vi "Dashboard Main.vi"() -> ()   [LabVIEW 2020]
uses:
  <vilib>/event_ctls.llb/eventvkey.ctl
  <vilib>/Rock Robotics/Network Tables/NT Read Numeric Array.vi
  <vilib>/Rock Robotics/WPI/Dashboard/WPI_DashboardLogging Global.vi
panel:
  in  "Graph4":string="Number"
  in  "Graph3":string="Number"
  in  "Graph2":string="Number"
  in  "Graph1":string="Number"
  in  "Camera Settings Right":T1={"Frame Rate"=30, "Compression"=30, "Size"=1, "DB Camera Config"=FALSE} {"Frame Rate" scale=1.0..30.0; "Compression" scale=100.0..-1.0; "Size" items=["640x480", "320x240", "160x120"]}
  in  "Camera Name Right":string(combo)="No Camera Selection"
  out "Camera Perf":string
  in  "Camera Settings":T1={"Frame Rate"=30, "Compression"=30, "Size"=1, "DB Camera Config"=FALSE} {"Frame Rate" scale=1.0..30.0; "Compression" scale=100.0..-1.0; "Size" items=["640x480", "320x240", "160x120"]}
  in  "TCP":refnum<k5>
  in  "Rec Mode":enum32{"Stop", "Record", "Playback"}(radio)
  out "Robot IP":string
  out "Image Message":string="Timeout in Camera Communications"
  in  "Dashboard Tab":T2(tab)
  out "Waveform Graph":dbl[](graph)
  in  "Select Auto":string(combo)="Select Autonomous ..."
  out "NT Connection":bool
  out "Mode":T3(ring)=enum."Auto Disabled"
  out "Right Camera Perf":cluster{"Bandwidth (Mbps)":dbl, "FPS":dbl}
  out "Camera Image Right":T4(plugin-control)
  in  "DB/String 9":string
  in  "DB/String 8":string
  in  "DB/String 7":string
  in  "DB/String 6":string
  in  "DB/String 5":string
  in  "DB/String 4":string
  in  "DB/String 3":string
  in  "DB/String 2":string
  in  "DB/String 1":string
  in  "DB/String 0":string
  in  "DB/Slider 0":dbl(slide) scale=0.0..5.0
  in  "DB/Slider 1":dbl(slide) scale=0.0..5.0
  in  "DB/Slider 2":dbl(slide) scale=0.0..5.0
  in  "DB/Slider 3":dbl(slide) scale=0.0..5.0
  out "DB/LED 3":bool
  out "DB/LED 2":bool
  out "DB/LED 1":bool
  out "DB/LED 0":bool
  in  "DB/Button 3":bool
  in  "DB/Button 2":bool
  in  "DB/Button 1":bool
  in  "DB/Button 0":bool caption="New Name"
  in  "Test Slider":dbl(slide) scale=0.0..100.0 scale format="%#_3g"
  in  "On/Off":bool caption="Solenoid"
  in  "Test Name":u16(ring) items=["Select the test to run..."]
  in  "Test Tree":string(tree)
  in  "Motor":cluster{"Value":dbl, "Enable":bool} {"Value" scale=-1.0..1.0 scale format="%#_3g"}
  out "Progress":T5 {"Test Progress" scale=0.0..100.0}
  in  "Rev/Fwd":cluster{"Forward":bool, "Reverse":bool}
  in  "Test Ring":u16(ring) items=["Monochrome", "Color"]
  in  "CheckList":i32(listbox)
  out "Tree":string(tree)
  out "Camera Image":T4(plugin-control)
  out "Background":bool
  in  "Camera Name":string(combo)="No Camera Selection"
  # "HW"
  # "HW"
  # "This tab is a great place for autonomous settings and robot-specific values.\nPlace controls and indicators inside this tab and match name to\nDashboard Variables on robot. You can also delete this comment."
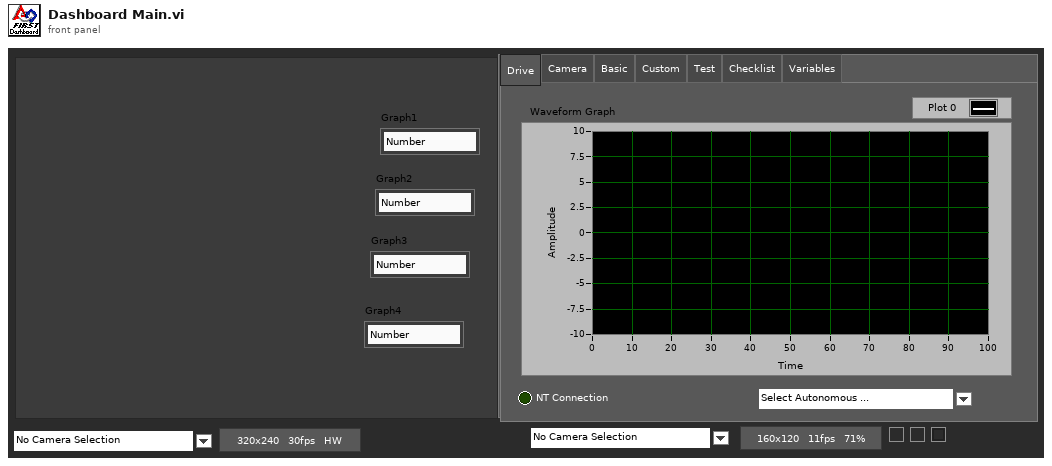
[diagram p1: front panel]
types:
  T1 = cluster{"Frame Rate":i32, "Compression":i32, "Size":u16, "DB Camera Config":bool}
  T2 = enum32{"Drive", "Camera", "Basic", "Custom", "Test", "Checklist", "Variables"}
  T3 = enum8{"Tele-Op Disabled", "Tele-Op Enabled", "Auto Disabled", "Auto Enabled", "Test Disabled", "Test Enabled", "Disconnected", "No Code", "E-Stop"}
  T4 = typedef "IMAQ Image.ctl" = refnum<image>
  T5 = cluster{"Test Progress":u8, "Test Progress Text":string}
  T6 = cluster{"Save Path":path, "Interval (s)":dbl, "Keep":i32}
  T7 = enum32{"Drive", "Camera", "Basic", "Custom", "Test", "Commands", "Checklist", "Variables"}
  T8 = typedef "Image Type" = u32
  T9 = cluster{"Error Strings":string, "Disable Counts":cluster{u16, u16}, "Rail Faults":cluster{u16, u16, u16}, "Robot IP":string, "DB Mode":u8, "Event Info":cluster{"Name":string, "Type":u8, "Number":u16, "Replay":u8}}
  T10 = cluster{"Storage":cluster{"Disk Free":u64, "RAM Block":u32, "RAM free":u32}, "CPU Utilization":cluster{"CPU % ISR":sgl, "CPU % Time Crit":sgl, "CPU % Timed Str":sgl, "CPU % High":sgl, "CPU % Above":sgl, "CPU % Normal":sgl, "CPU % Low":sgl}, "CAN":cluster{"% Bus Utilization":sgl, "Bus Off Cnt":u32, "TX_FIFO Full Cnt":u32, "Receive Error Cnt":u8, "Transmit Error Cnt":u8}, "HID":cluster{"HID Outputs":u32, "Rumble Low":u16, "Rumble High":u16}[]}
  T11 = cluster{"Status bits":cluster{"Test Mode":bool, "Autonomous":bool, "Enabled":bool, "Code Start":bool, "Brownout":bool, "Reserved 2":bool, "Reserved 3":bool, "E-Stop":bool}, "Code Trace":cluster{"Disabled":bool, "TeleOp":bool, "Auto":bool, "Test":bool}, "Controller Type":enum16{"unknown", "cRIO", "roboRio"}, "Code?":enum16{"unknown", "noCode", "code"}, "Battery V":dbl}
  T12 = cluster{"Control Bits":cluster{"TestMode":bool, "Autonomous":bool, "Enabled":bool, "FMS Present":bool, bool, bool, bool, "E-Stop":bool}, "Team Station ":u8, "Countdown":sgl, "Joystick Values":cluster{"Axes":dbl[], "Buttons":bool[], "POVs":i16[]}[]}
  T13 = cluster{"Axes":dbl[], "Buttons":bool[], "POVs":i16[]}[]
  T14 = cluster{"Axes":dbl[], "Buttons":bool[], "POVs":i16[]}
  T15 = cluster{"Camera Image":refnum<vi>, "Dashboard Tab":refnum<vi>, "Background":refnum<vi>, "Rec Mode":refnum<vi>, "Test Slider":refnum<vi>, "On/Off ":refnum<vi>, "Test Ring":refnum<vi>, "Rev/Fwd":refnum<vi>, "Test Name":refnum<vi>, "Motor":refnum<vi>, "Progress":refnum<vi>, "CheckList":refnum<vi>, "Tree":refnum<vi>, "Test Tree":refnum<vi>, "Camera Settings":refnum<vi>, "Camera Name":refnum<vi>, "Camera Perf":refnum<vi>, "Camera Settings Right":refnum<vi>, "Camera Name Right":refnum<vi>, "Camera Image Right":refnum<vi>}
  T16 = cluster{"Global Rectangle":i32[], "Contours":cluster{"Contour Type":u32, "ROI Type":u32, "Points":i32[]}[]}
  T17 = cluster{"Camera Name":string, string, "Saved DB Images Info":cluster{"Save Path":path, "Interval (s)":dbl, "Keep":i32}}
  T18 = cluster{"Camera Name Right":string, string, "Saved DB Images Info":cluster{"Save Path":path, "Interval (s)":dbl, "Keep":i32}}
  T19 = cluster{"Operation":enum16{"Update", "Clear"}, "Color Box":u32}[]
  T20 = typedef "eventvkey.ctl" = enum16{"ASCII", "Enter", "Return", "Shift", "Ctrl", "Alt", "Cmd", "Opt", "Caps", "NumLock", "Clear", "Break", "Up", "Down", "Left", "Right", "Insert", "Delete", "Home", "End", "PageUp", "PageDown", "Escape", "Help", "Pause", "ScrollLock", "F1", "F2", "F3", "F4", "F5", "F6", "F7", "F8", "F9", "F10", "F11", "F12", "F13", "F14", "F15", "F16", "F17", "F18", "F19", "F20", "F21", "F22", "F23", "F24", "Play", "VolumeUp", "VolumeDown", "Mute", "Two Byte Char"}
  T21 = cluster{"Image Size":bool, "Image Type":bool, "Pixel Value":bool, "ROI Information":bool, "Zoom Factor":bool}
  T22 = cluster{"Operation":enum16{"Update", "Clear"}, "Color Box":u32}
  T23 = cluster{"Shift":bool, "Ctrl":bool, "Alt":bool, "Cmd":bool, "Opt":bool}
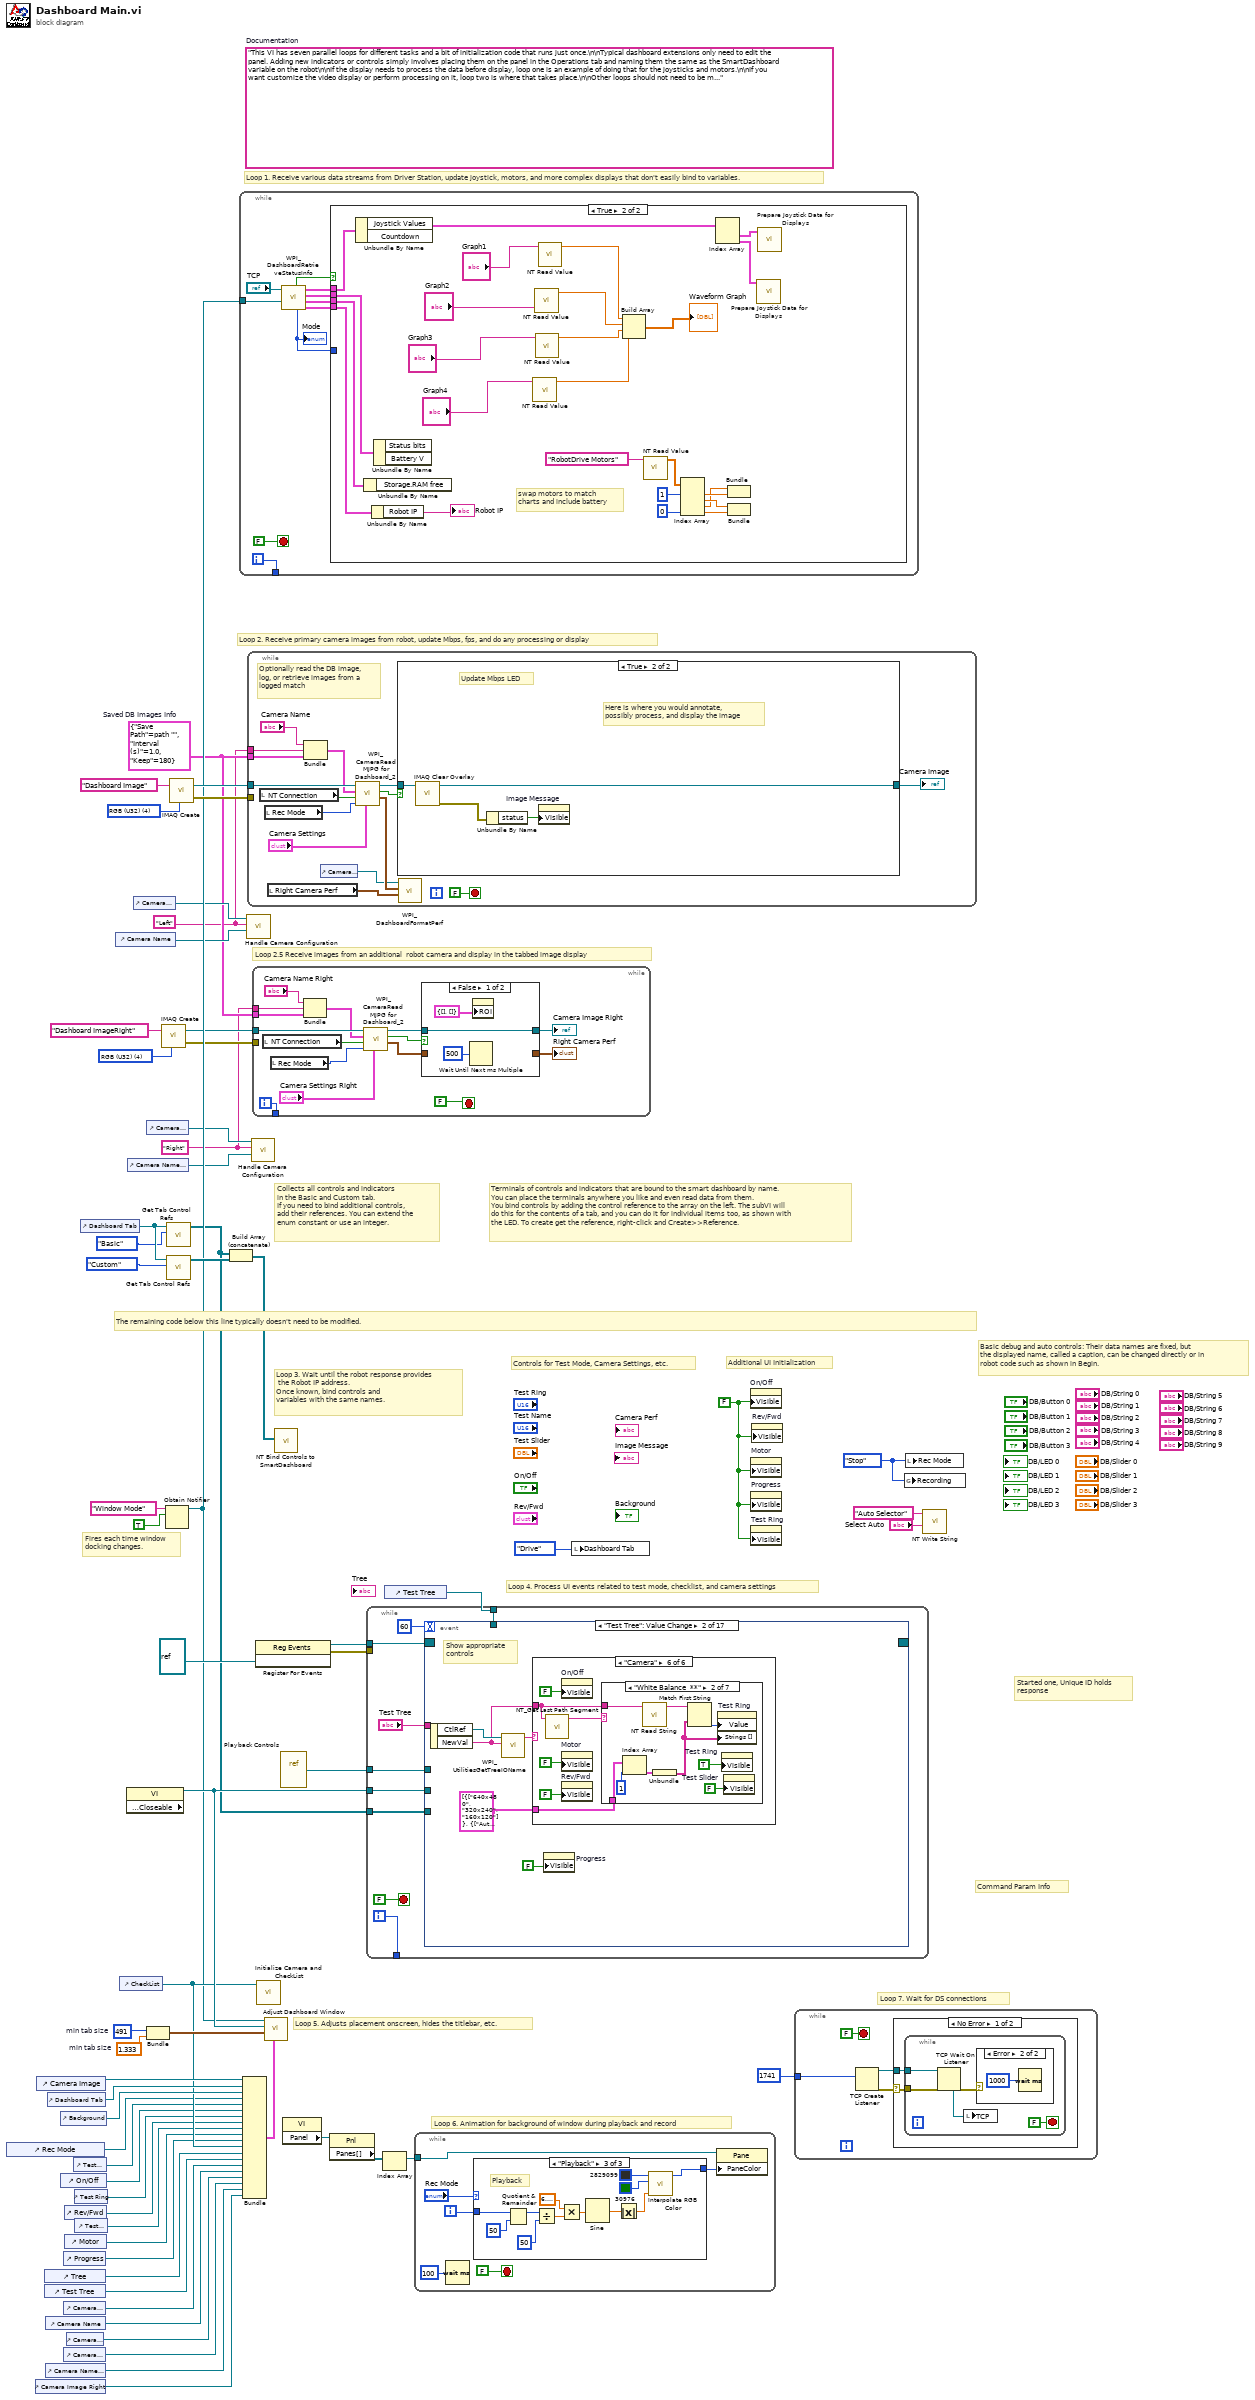
[diagram p0: block diagram]
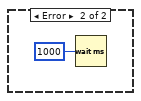
[diagram p4: hidden frame]
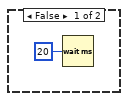
[diagram p5: hidden frame]
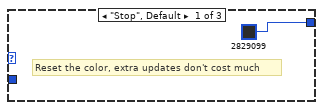
[diagram p6: hidden frame]
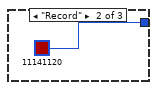
[diagram p7: hidden frame]
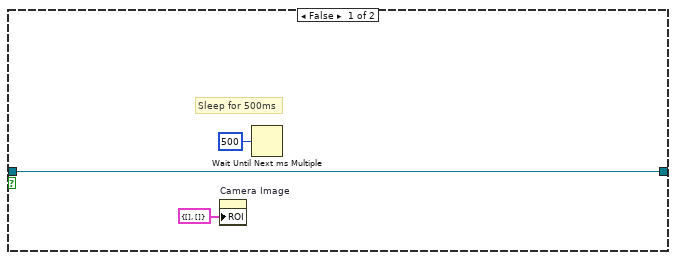
[diagram p8: hidden frame]
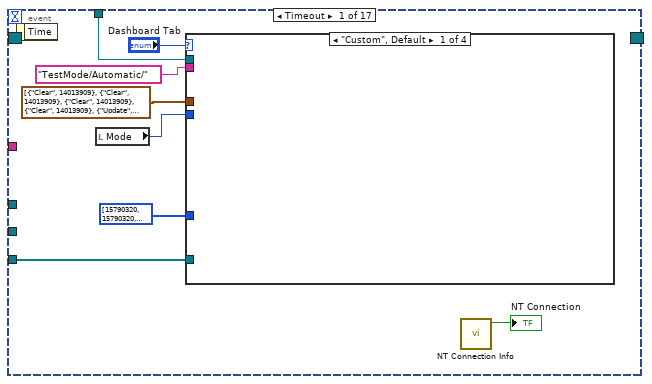
[diagram p9: hidden frame]
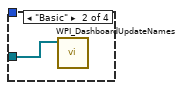
[diagram p10: hidden frame]
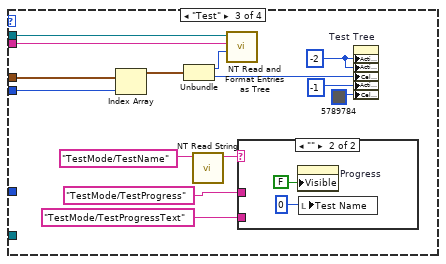
[diagram p11: hidden frame]
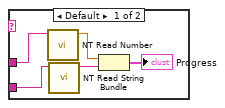
[diagram p12: hidden frame]
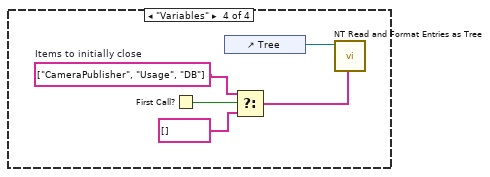
[diagram p13: hidden frame]
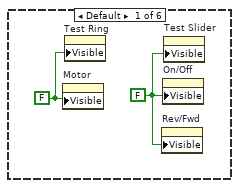
[diagram p14: hidden frame]
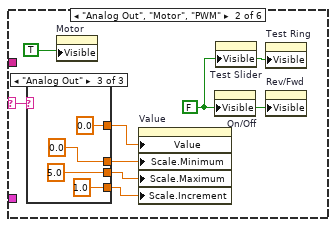
[diagram p15: hidden frame]
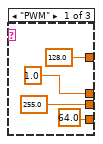
[diagram p16: hidden frame]
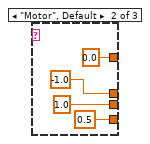
[diagram p17: hidden frame]
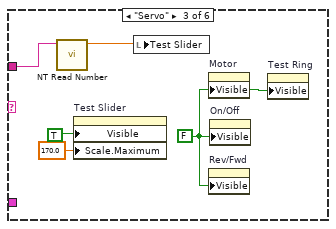
[diagram p18: hidden frame]
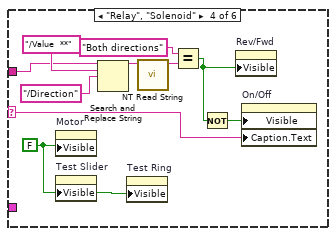
[diagram p19: hidden frame]
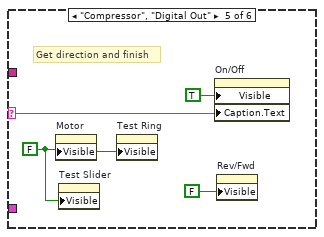
[diagram p20: hidden frame]
diagram:
  w3 = T6 {"Save Path"=path "", "Interval (s)"=1.0, "Keep"=180}  # Saved DB Images Info
  w2 = "Right"
  w1 = "Left"
  w13 = T8 4 items=["Grayscale (U8)", "Grayscale (I16)", "Grayscale (SGL)", "Complex (CSG)", "RGB (U32)", "HSL (U32)", "RGB (U64)"] ("Image Type")
  w42 = 491  # min tab size
  w41 = 1.333  # min tab size
  w49 = enum32{"Stop", "Record", "Playback"}."Stop" ("Rec Mode")
  w26 = FALSE ("Visible")
  (unwired) "This VI has seven parallel loops for different tasks and a bit of initialization code that runs just once.\n\nTypical dashboard extensions only need to edit the panel. Adding new indicators or controls simply involves placing them on the panel in the Operations tab and naming them the same as the SmartDashboard variable on the robot\n\nIf the display needs to process the data before display, loop one is an example of doing that for the joysticks and motors.\n\nIf you want customize the video display or perform processing on it, loop two is where that takes place.\n\nOther loops should not need to be modified. They are pretty standard, and document the task they perform."  # Documentation
  w63 = T8 4 items=["Grayscale (U8)", "Grayscale (I16)", "Grayscale (SGL)", "Complex (CSG)", "RGB (U32)", "HSL (U32)", "RGB (U64)"] ("Image Type")
  # "Loop 2.5 Receive images from an additional  robot camera and display in the tabbed image display"
  # "Command Param Info"
  # "Started one, Unique ID holds\nresponse"
  # "Loop 7. Wait for DS connections"
  # "Basic debug and auto controls: Their data names are fixed, but\nthe displayed name, called a caption, can be changed directly or in\nrobot code such as shown in Begin."
  # "Controls for Test Mode, Camera Settings, etc."
  # "Additional UI Initialization"
  # "Loop 6. Animation for background of window during playback and record"
  # "Fires each time window\ndocking changes."
  # "Collects all controls and indicators\nin the Basic and Custom tab.\nIf you need to bind additional controls,\nadd their references. You can extend the\nenum constant or use an integer."
  # "The remaining code below this line typically doesn't need to be modified."
  # "Loop 4. Process UI events related to test mode, checklist, and camera settings"
  # "Terminals of controls and indicators that are bound to the smart dashboard by name.\nYou can place the terminals anywhere you like and even read data from them.\nYou bind controls by adding the control reference to the array on the left. The subVI will\ndo this for the contents of a tab, and you can do it for individual items too, as shown with\nthe LED. To create get the reference, right-click and Create>>Reference."
  # "Loop 3. Wait until the robot response provides\n the Robot IP address.\nOnce known, bind controls and\nvariables with the same names."
  # "Loop 5. Adjusts placement onscreen, hides the titlebar, etc."
  # "Loop 1. Receive various data streams from Driver Station, update joystick, motors, and more complex displays that don't easily bind to variables."
  # "Loop 2. Receive primary camera images from robot, update Mbps, fps, and do any processing or display"
  n1 = control-ref of="Rec Mode"() -> (w32:refnum<vi>)
  n2 = control-ref of="Camera Image Right"() -> (w6:refnum<vi>)
  n3 = control-ref of="Camera Image"() -> (w44:refnum<vi>)
  n4 = control-ref of="Tree"() -> (w36:refnum<vi>)
  n5 = control-ref of="Test Tree"() -> (w35:refnum<vi>)
  n6 = control-ref of="Camera Name"() -> (w19:refnum<vi>)
  n7 = control-ref of="Camera Name Right"() -> (w7:refnum<vi>)
  n8 = control-ref of="Dashboard Tab"() -> (w43:refnum<vi>)
  n9 = control-ref of="Background"() -> (w39:refnum<vi>)
  n10 = control-ref of="On/Off"() -> (w30:refnum<vi>)
  n11 = control-ref of="Progress"() -> (w27:refnum<vi>)
  n12 = control-ref of="Camera Settings"() -> (w20:refnum<vi>)
  n13 = control-ref of="Camera Settings Right"() -> (w8:refnum<vi>)
  n14 = control-ref of="Rev/Fwd"() -> (w28:refnum<vi>)
  n15 = control-ref of="Motor"() -> (w33:refnum<vi>)
  n16 = control-ref of="Camera Perf"() -> (w18:refnum<vi>)
  n17 = control-ref of="Test Slider"() -> (w31:refnum<vi>)
  n18 = control-ref of="Test Ring"() -> (w29:refnum<vi>)
  n19 = control-ref of="Test Name"() -> (w34:refnum<vi>)
  n20 = control-ref of="Dashboard Tab"() -> (w47:refnum<vi>)
  n21 = control-ref of="Camera Name"() -> (w21:refnum<vi>)
  n22 = control-ref of="CheckList"() -> (w37:refnum<vi>)
  n23 = property class="VI" props=["Front Panel.Closeable"]() -> (reference out=w48:refnum<vi>)  [unwired: 2 in, 2 out]
  n24 = control-ref of="Camera Name Right"() -> (w9:refnum<vi>)
  n25 = control-ref of="Camera Settings"() -> (w22:refnum<vi>)
  n26 = control-ref of="Camera Settings Right"() -> (w10:refnum<vi>)
  n27 = Bundle("min tab size"=w42, "min tab size"=w41) -> (w40:cluster{"min tab size":i32, "min tab size":dbl})  [unwired: 1 in]
  n28 = call "IMAQ Create"("Image Name"="Dashboard ImageRight", "Image Type"=w13) -> ("New Image"=w12:T4, "error out"=w11:errorcluster)  [unwired: 2 in, 1 out]
  n29 = Obtain Notifier(name (unnamed)="Window Mode", notification data type=TRUE) -> (notifier out=w25:refnum<notifier>)  [unwired: 2 in, 2 out]
  n30 = call <vilib>:"Get Tab Control Refs.vi"("Page Index"=T7."Basic" ("Dashboard Tab"), "TabControl in"=w47) -> ("ControlsOnPage"=w17:refnum<vi>[])  [unwired: 9 in]
  n31 = call <vilib>:"Get Tab Control Refs.vi"("Page Index"=T7."Custom" ("Dashboard Tab"), "TabControl in"=w47) -> ("ControlsOnPage"=w46:refnum<vi>[])  [unwired: 9 in]
  n32 = call "IMAQ Create"("Image Name"="Dashboard Image", "Image Type"=w63) -> ("New Image"=w61:T4, "error out"=w60:errorcluster)  [unwired: 2 in, 1 out]
  n33 = Build Array (concatenate)(w17, w46) -> (w45:refnum<vi>[])
  n34 = while {
    tunnel: [w72] -> _
    tunnel: w25 -> [w64]
    i -> [w72]
    stop <- FALSE stop-if-true
    n35 = call <vilib>:"WPI_DashboardRetrieveStatusInfo.vi"("Window Mode Notifier"=w64, "TCP Cnx"="TCP") -> ("Power and Errors"=w67:T9, "Robot Metrics"=w70:T10, "Status Info"=w71:T11, "Control Info"=w68:T12, "Robot Mode"=w66:T3, "Process?"=w69:bool)  [unwired: 4 in]
    "Mode" <- w66
    n36 = case shown="True" w69 {
      tunnel: w71 -> [_ w99]
      tunnel: w70 -> [_ w98]
      tunnel: w68 -> [_ w97]
      tunnel: w67 -> [_ w96]
      tunnel: w66 -> [_ _]
      frame False {
        n37 = Wait (ms)(milliseconds to wait=u32 20) -> ()  [unwired: 1 out]
      }
      frame True {
        # "swap motors to match\ncharts and include battery"
        n38 = Unbundle By Name(w97) -> ("Joystick Values"=w89:T13)  [unwired: 1 out]
        n39 = Unbundle By Name(w98) -> ()  [unwired: 1 out]
        n40 = Unbundle By Name(w96) -> ("Robot IP"=→"Robot IP":string)
        n41 = Unbundle By Name(w99) -> ()  [unwired: 2 out]
        n42 = call-poly <vilib>:"NT Read Value.vi"("name"="Graph4") -> ("value"=w79:dbl)  [unwired: 8 in, 2 out]
        n43 = call-poly <vilib>:"NT Read Value.vi"("name"="Graph2") -> ("value"=w81:dbl)  [unwired: 8 in, 2 out]
        n44 = call-poly <vilib>:"NT Read Value.vi"("name"="Graph3") -> ("value"=w80:dbl)  [unwired: 8 in, 2 out]
        n45 = call-poly <vilib>:"NT Read Value.vi"("name"="Graph1") -> ("value"=w82:dbl)  [unwired: 8 in, 2 out]
        n46 = Build Array(w82, w81, w80, w79) -> (→"Waveform Graph":dbl[])
        n47 = call-poly <vilib>:"NT Read Value.vi"("name"="RobotDrive Motors" ("Name")) -> ("value"=w85:dbl[])  [unwired: 8 in, 2 out]
        n48 = Index Array(array=w85, index #1=1, index #4=0) -> (element #1=w91:dbl, element #2=w92:dbl, element #3=w90:dbl, element #4=w95:dbl)  [unwired: 2 in]
        n49 = Index Array(array=w89) -> (element #1=w88:T14, element #2=w87:T14)  [unwired: 2 in]
        n50 = Bundle("Numeric"=w90, "Numeric"=w91) -> ()  [unwired: 1 in, 1 out]
        n51 = Bundle("Numeric"=w92, "Numeric"=w95) -> ()  [unwired: 1 in, 1 out]
        n52 = call "Prepare Joystick Data for Displays.vi"("Joystick Values"=w87) -> ()  [unwired: 8 in, 3 out]
        n53 = call "Prepare Joystick Data for Displays.vi"("Joystick Values"=w88) -> ()  [unwired: 8 in, 3 out]
      }
    }
  }
  n54 = Bundle("Camera Image"=w44, "Dashboard Tab"=w43, "Background"=w39, "Rec Mode"=w32, "Test Slider"=w31, "On/Off"=w30, "Test Ring"=w29, "Rev/Fwd"=w28, "Test Name"=w34, "Motor"=w33, "Progress"=w27, "CheckList"=w37, "Tree"=w36, "Test Tree"=w35, "Camera Settings"=w20, "Camera Name"=w19, "Camera Perf"=w18, "Camera Settings Right"=w8, "Camera Name Right"=w7, "Camera Image Right"=w6) -> (w38:T15)  [unwired: 1 in]
  n55 = call "Handle Camera Configuration.vi"("CameraNameRef"=w21, "Display Name"=w1, "ClusterRef"=w22) -> ()  [unwired: 9 in]
  n56 = while {
    tunnel: w61 -> [w113]
    tunnel: w60 -> [_]
    tunnel: w3 -> [w106]
    tunnel: w1 -> [w103]
    stop <- FALSE stop-if-true
    # "Optionally read the DB image,\nlog, or retrieve images from a\nlogged match"
    n57 = local read "NT Connection"() -> (w107:bool)
    n58 = local read "Rec Mode"() -> (w110:enum32{"Stop", "Record", "Playback"})
    n59 = local read "Right Camera Perf"() -> (w101:cluster{"Bandwidth (Mbps)":dbl, "FPS":dbl})
    n60 = Bundle("Camera Name"="Camera Name", w103, "Saved DB Images Info"=w106) -> (w105:T17)  [unwired: 1 in]
    n61 = control-ref of="Camera Perf"() -> (w100:refnum<vi>)
    n62 = call <vilib>:"WPI_CameraRead MJPG for Dashboard_2.vi"("Camera Settings"="Camera Settings", "Rec Mode"=w110, "NT Connection"=w107, "Capture Info"=w105, "Image in"=w113) -> ("perf info"=w102:cluster{"Bandwidth (Mbps)":dbl, "fps":dbl}, "Active"=w111:bool, "Image\\ out"=w112:T4)  [unwired: 4 in]
    n63 = case shown="True" w111 {
      tunnel: w112 -> [w116 w119]
      tunnel: [w116 w118] -> w108
      frame False {
        # "Sleep for 500ms"
        n64 = property on="Camera Image" class="ImageControl"("ROI"=T16 {"Global Rectangle"=[], "Contours"=[]}) -> ()  [unwired: 2 in, 2 out]
        n65 = Wait Until Next ms Multiple(millisecond multiple=u32 500) -> ()  [unwired: 1 out]
      }
      frame True {
        # "Here is where you would annotate,\npossibly process, and display the image"
        # "Update Mbps LED"
        n66 = call "IMAQ Clear Overlay"("Image"=w119) -> ("error out"=w120:errorcluster, "Image Out"=w118:T4)  [unwired: 2 in, 7 out]
        n67 = Unbundle By Name(w120) -> ("status"=w121:bool)
        n68 = property on="Image Message" class="Str"("Visible"=w121) -> ()  [unwired: 2 in, 2 out]
      }
    }
    "Camera Image" <- w108
    n69 = call <vilib>:"WPI_DashboardFormatPerf.vi"("Right Camera Perf"=w101, "Performance"=w102, "String in"=w100) -> ()  [unwired: 9 in]
  }
  n70 = call "Handle Camera Configuration.vi"("CameraNameRef"=w9, "Display Name"=w2, "ClusterRef"=w10) -> ()  [unwired: 9 in]
  n71 = while {
    tunnel: w12 -> [w136]
    tunnel: w11 -> [_]
    tunnel: [w131] -> _
    tunnel: w3 -> [w127]
    tunnel: w2 -> [w124]
    i -> [w131]
    stop <- FALSE stop-if-true
    n72 = local read "NT Connection"() -> (w128:bool)
    n73 = local read "Rec Mode"() -> (w135:enum32{"Stop", "Record", "Playback"})
    n74 = Bundle("Camera Name Right"="Camera Name Right", w124, "Saved DB Images Info"=w127) -> (w126:T18)  [unwired: 1 in]
    n75 = call <vilib>:"WPI_CameraRead MJPG for Dashboard_2.vi"("Camera Settings"="Camera Settings Right", "Rec Mode"=w135, "NT Connection"=w128, "Capture Info"=w126, "Image in"=w136) -> ("perf info"=w122:cluster{"Bandwidth (Mbps)":dbl, "fps":dbl}, "Active"=w130:bool, "Image\\ out"=w133:T4)  [unwired: 4 in]
    n76 = case shown="False" w130 {
      tunnel: w133 -> [w138 w141]
      tunnel: [w138 w141] -> w129
      tunnel: [_ w140] -> w123
      tunnel: w122 -> [_ w140]
      frame False {
        n77 = Wait Until Next ms Multiple(millisecond multiple=u32 500) -> ()  [unwired: 1 out]
        n78 = property on="Camera Image Right" class="ImageControl"("ROI"=T16 {"Global Rectangle"=[], "Contours"=[]}) -> ()  [unwired: 2 in, 2 out]
      }
      frame True {
      }
    }
    "Camera Image Right" <- w129
    "Right Camera Perf" <- w123
  }
  n79 = register-events(refnum<vi> refnum) -> (reference out=w52:refnum<event-registration>, error out=w51:errorcluster)  [unwired: 2 in]
  n80 = call "Initialize Camera and CheckList.vi"("ListBox in"=w37) -> ()  [unwired: 11 in]
  n81 = call "Adjust Dashboard Window.vi"("Sizing Refnums"=w38, "Size Constraints"=w40, "VI"=w48, "WIn Mode"=w25) -> ()  [unwired: 8 in]
  n82 = call <vilib>:"NT Bind Controls to SmartDashboard.vi"("Bound Control Refs"=w45) -> ()  [unwired: 11 in]
  n83 = vi-ref "Playback Controls.vi"() -> (w53:refnum<vi>)
  n84 = property class="VI"() -> ("Panel"=w55:refnum<vi>)  [unwired: 2 in, 2 out]
  n85 = property class="Pnl"(reference=w55) -> ("Panes[]"=w56:refnum<vi>[])  [unwired: 1 in, 2 out]
  n86 = Index Array(array=w56) -> (element=w54:refnum<vi>)  [unwired: 1 in]
  n87 = control-ref of="Test Tree"() -> (w57:refnum<vi>)
  n88 = while {
    tunnel: [w147] -> _
    tunnel: w57 -> [w146]
    tunnel: w53 -> [w145]
    tunnel: w52 -> [w144]
    tunnel: w51 -> [_]
    tunnel: w48 -> [w143]
    tunnel: w17 -> [w142]
    i -> [w147]
    stop <- FALSE stop-if-true
    n89 = event shown="[1] \"Test Tree\": Value Change" {
      selector: w144 -> [_ _ _ _ _ _ _ _ _ _ _ _ _ _ _ _ _]
      dyn-events: [_ _ _ _ _ _ _ _ _ _ _ _ _ w352 _ _ _] -> _
      timeout: u32 60 ("milliseconds to wait") -> [_ _ _ _ _ _ _ _ _ _ _ _ _ _ _ _ _]
      tunnel: w146 -> [w157 _ _ _ _ _ _ _ _ _ _ _ _ _ _ _ _]
      tunnel: "Test Tree" -> [_ _ _ _ _ _ _ _ w325 w332 w333 w336 w343 _ _ _ _]
      tunnel: w145 -> [_ _ _ _ _ _ _ _ _ _ _ _ _ w354 _ w369 _]
      tunnel: w143 -> [_ _ _ _ _ _ _ _ _ _ _ _ _ w350 _ _ _]
      tunnel: w142 -> [w152 _ _ _ _ _ _ _ _ _ _ _ _ _ _ _ _]
      event Timeout {
        n90 = event-data() -> ()  [unwired: 1 in, 1 out]
        n91 = local read "Mode"() -> (w155:T3)
        n92 = case shown="\"Custom\", Default" "Dashboard Tab" {
          tunnel: w157 -> [_ _ w173 _]
          tunnel: "TestMode/Automatic/" ("Name Pattern") -> [_ _ w172 _]
          tunnel: T19 [{"Operation"=enum."Clear", "Color Box"=14013909}, {"Operation"=enum."Clear", "Color Box"=14013909}, {"Operation"=enum."Clear", "Color Box"=14013909}, {"Operation"=enum."Clear", "Color Box"=14013909}, {"Operation"=enum."Update", "Color Box"=14013909}, {"Operation"=enum."Update", "Color Box"=16777215}, {"Operation"=enum."Clear", "Color Box"=14013909}, {"Operation"=enum."Clear", "Color Box"=14013909}, {"Operation"=enum."Clear", "Color Box"=14013909}] -> [_ _ w165 _]
          tunnel: w155 -> [_ _ w164 _]
          tunnel: u32[] [15790320, 15790320, 15790320, 15790320, 16777215, 16777215, 15790320, 15790320, 15790320] -> [_ _ _ _]
          tunnel: w152 -> [_ w159 _ _]
          frame "Custom", Default {
          }
          frame "Basic" {
            n93 = call <vilib>:"WPI_DashboardUpdateNames.vi"("Controls on Tab"=w159) -> ()  [unwired: 11 in]
          }
          frame "Test" {
            w171 = -2 ("Active Item:Row Number")
            n94 = Index Array(array=w165, index=w164) -> (element=w166:T22)
            n95 = Unbundle(w166) -> ("Operation"=w167:enum16{"Update", "Clear"}, "Color Box"=w168:u32)
            n96 = call <vilib>:"NT Read String.vi"("name"="TestMode/TestName" ("Name")) -> ("value"=w162:string)  [unwired: 8 in, 2 out]
            n97 = call <vilib>:"NT Read and Format Entries as Tree.vi"("Operation"=w167, "Name Pattern"=w172, "Tree Refnum"=w173) -> ()  [unwired: 7 in, 2 out]
            n98 = case shown="\"\"" w162 {
              tunnel: "TestMode/TestProgress" ("Name") -> [w175 _]
              tunnel: "TestMode/TestProgressText" ("Name") -> [w174 _]
              frame Default {
                n99 = call <vilib>:"NT Read Number.vi"("name"=w175) -> ("value"=w176:dbl)  [unwired: 8 in, 2 out]
                n100 = call <vilib>:"NT Read String.vi"("name"=w174) -> ("value"=w177:string)  [unwired: 8 in, 2 out]
                n101 = Bundle("value"=w176, "value"=w177) -> (→"Progress":cluster{"value":dbl, "value":string})  [unwired: 1 in]
              }
              frame "" {
                n102 = property on="Progress" class="Clust (strict)"("Visible"=FALSE) -> ()  [unwired: 2 in, 2 out]
                n103 = local write "Test Name"(u16 0) -> ()
              }
            }
            n104 = property on="Test Tree" class="Tree (strict)"("Active Item Row Number"=w171, "ActiveColNum"=w171, "CellBG"=w168, "Active Item Row Number"=-1 ("Active Item:Row Number"), "CellBG"=u32 5789784 ("Color Box")) -> ()  [unwired: 2 in, 2 out]
          }
          frame "Variables" {
            w183 = string[] ["CameraPublisher", "Usage", "DB"]  # Items to initially close
            n105 = First Call?() -> (First Call?: T/F=w184:bool)
            n106 = control-ref of="Tree"() -> (w185:refnum<vi>)
            n107 = Select(t=w183, s=w184, f=string[] []) -> (s? t:f=w181:string[])
            n108 = call <vilib>:"NT Read and Format Entries as Tree.vi"("Tags to  Close"=w181, "Tree Refnum"=w185) -> ()  [unwired: 8 in, 2 out]
          }
        }
        n109 = call <vilib>:"NT Connection Info.vi"() -> ("Connected"=→"NT Connection":bool)  [unwired: 11 in]
      }
      event "Test Tree": Value Change {
        # "Show appropriate\ncontrols"
        n110 = event-data() -> ("CtlRef"=w189:refnum<vi>, "NewVal"=w187:string)  [unwired: 1 in]
        n111 = call <vilib>:"WPI_UtilitiesGetTreeIOName.vi"("NewVal"=w187, "TreeControl in"=w189) -> ("I/O Name"=w190:string)  [unwired: 9 in]
        n112 = case shown="\"Camera\"" w190 {
          selector: w190 -> [_ w197 _ w219 w228 _]
          tunnel: w187 -> [_ _ w216 w218 _ w235]
          tunnel: cluster{string[]}[] [{["640x480", "320x240", "160x120"]}, {["Auto", "Fixed indoor", "Fixed outdoor 1", "Fixed outdoor 2", "Fixed fluorescent 1", "Fixed fluorescent 2", "Hold current"]}, {["Auto", "Flicker-free 50 Hz", "Flicker-free 60 Hz", "Hold current"]}, {["None", "Prioritize frame rate", "Prioritize image quality"]}, {["Monochrome", "Color"]}] -> [_ _ _ _ _ w234]
          frame Default {
            w192 = FALSE ("Visible")
            w191 = FALSE ("Visible")
            n113 = property on="Motor" class="Clust (strict)"("Visible"=w191) -> ()  [unwired: 2 in, 2 out]
            n114 = property on="Test Ring" class="Ring (strict)"("Visible"=w191) -> ()  [unwired: 2 in, 2 out]
            n115 = property on="Rev/Fwd" class="Clust (strict)"("Visible"=w192) -> ()  [unwired: 2 in, 2 out]
            n116 = property on="On/Off" class="Bool (strict)"("Visible"=w192) -> ()  [unwired: 2 in, 2 out]
            n117 = property on="Test Slider" class="Slide (strict)"("Visible"=w192) -> ()  [unwired: 2 in, 2 out]
          }
          frame "Analog Out", "Motor", "PWM" {
            w198 = FALSE ("Visible")
            n118 = case shown="\"Analog Out\"" w197 {
              tunnel: [1.0 ("Value") -1.0 ("Value") 0.0 ("Value")] -> w196
              tunnel: [255.0 ("Value") 1.0 ("Value") 5.0 ("Value")] -> w195
              tunnel: [128.0 ("Value") 0.0 ("Value") 0.0 ("Value")] -> w194
              tunnel: [64.0 ("Value") 0.5 ("Value") 1.0 ("Value")] -> w193
              frame "PWM" {
              }
              frame "Motor", Default {
              }
              frame "Analog Out" {
              }
            }
            n119 = property on="Motor" class="Clust (strict)"("Visible"=TRUE) -> ()  [unwired: 2 in, 2 out]
            n120 = property on="Value" class="Slide (strict)"("Value"=w194, "Scale.Minimum"=w196, "Scale.Maximum"=w195, "Scale.Increment"=w193) -> ()  [unwired: 2 in, 2 out]
            n121 = property on="On/Off" class="Bool (strict)"("Visible"=w198) -> ()  [unwired: 2 in, 2 out]
            n122 = property on="Test Slider" class="Slide (strict)"("Visible"=w198) -> ()  [unwired: 2 in, 2 out]
            n123 = property on="Test Ring" class="Ring (strict)"("Visible"=w198) -> ()  [unwired: 2 in, 2 out]
            n124 = property on="Rev/Fwd" class="Clust (strict)"("Visible"=w198) -> ()  [unwired: 2 in, 2 out]
          }
          frame "Servo" {
            w214 = FALSE ("Visible")
            n125 = call <vilib>:"NT Read Number.vi"("name"=w216) -> ("value"=w215:dbl)  [unwired: 8 in, 2 out]
            n126 = property on="Test Slider" class="Slide (strict)"("Visible"=TRUE, "Scale.Maximum"=170.0 ("Scale.Range:Maximum")) -> ()  [unwired: 2 in, 2 out]
            n127 = local write "Test Slider"(w215) -> ()
            n128 = property on="Motor" class="Clust (strict)"("Visible"=w214) -> ()  [unwired: 2 in, 2 out]
            n129 = property on="Rev/Fwd" class="Clust (strict)"("Visible"=w214) -> ()  [unwired: 2 in, 2 out]
            n130 = property on="On/Off" class="Bool (strict)"("Visible"=w214) -> ()  [unwired: 2 in, 2 out]
            n131 = property on="Test Ring" class="Ring (strict)"("Visible"=w214) -> ()  [unwired: 2 in, 2 out]
          }
          frame "Relay", "Solenoid" {
            w217 = FALSE ("Visible")
            n132 = property on="Motor" class="Clust (strict)"("Visible"=w217) -> ()  [unwired: 2 in, 2 out]
            n133 = property on="Test Slider" class="Slide (strict)"("Visible"=w217) -> ()  [unwired: 2 in, 2 out]
            n134 = Search and Replace String(input string=w218, search string="/Value  **", replace string="/Direction") -> (result string=w224:string)  [unwired: 5 in, 3 out]
            n135 = property on="Test Ring" class="Ring (strict)"("Visible"=w217) -> ()  [unwired: 2 in, 2 out]
            n136 = call <vilib>:"NT Read String.vi"("name"=w224) -> ("value"=w222:string)  [unwired: 8 in, 2 out]
            n137 = Equal?(x="Both directions", y=w222) -> (x = y?=w220:bool)
            n138 = Not(x=w220) -> (.not. x?=w221:bool)
            n139 = property on="Rev/Fwd" class="Clust (strict)"("Visible"=w220) -> ()  [unwired: 2 in, 2 out]
            n140 = property on="On/Off" class="Bool (strict)"("Visible"=w221, "Caption.Text"=w219) -> ()  [unwired: 2 in, 2 out]
          }
          frame "Compressor", "Digital Out" {
            w227 = FALSE ("Visible")
            # "Get direction and finish"
            n141 = property on="Motor" class="Clust (strict)"("Visible"=w227) -> ()  [unwired: 2 in, 2 out]
            n142 = property on="Test Slider" class="Slide (strict)"("Visible"=w227) -> ()  [unwired: 2 in, 2 out]
            n143 = property on="Test Ring" class="Ring (strict)"("Visible"=w227) -> ()  [unwired: 2 in, 2 out]
            n144 = property on="On/Off" class="Bool (strict)"("Visible"=TRUE, "Caption.Text"=w228) -> ()  [unwired: 2 in, 2 out]
            n145 = property on="Rev/Fwd" class="Clust (strict)"("Visible"=FALSE) -> ()  [unwired: 2 in, 2 out]
          }
          frame "Camera" {
            n146 = call <vilib>:"NT_Get Last Path Segment.vi"("String in"=w235) -> ("String out"=w236:string)  [unwired: 10 in]
            n147 = property on="On/Off" class="Bool (strict)"("Visible"=FALSE) -> ()  [unwired: 2 in, 2 out]
            n148 = property on="Motor" class="Clust (strict)"("Visible"=FALSE) -> ()  [unwired: 2 in, 2 out]
            n149 = property on="Rev/Fwd" class="Clust (strict)"("Visible"=FALSE) -> ()  [unwired: 2 in, 2 out]
            n150 = case shown="\"White Balance  **\"" w236 {
              tunnel: w235 -> [w242 w251 w260 w269 w278 _ w284]
              tunnel: w234 -> [w240 w248 w257 w266 w275 _ _]
              frame "Size  **" {
                n151 = Index Array(array=w240) -> (element=w239:cluster{string[]})  [unwired: 1 in]
                n152 = call <vilib>:"NT Read String.vi"("name"=w242) -> ("value"=w241:string)  [unwired: 8 in, 2 out]
                n153 = Unbundle(w239) -> (w237:string[])
                n154 = Match First String(2:w237, 3:w241) -> (0:w238:i32)  [unwired: 1 out]
                n155 = property on="Test Ring" class="Ring (strict)"("Value"=w238, "Strings []"=w237) -> ()  [unwired: 2 in, 2 out]
                n156 = property on="Test Ring" class="Ring (strict)"("Visible"=TRUE) -> ()  [unwired: 2 in, 2 out]
                n157 = property on="Test Slider" class="Slide (strict)"("Visible"=FALSE) -> ()  [unwired: 2 in, 2 out]
              }
              frame "White Balance  **" {
                n158 = Index Array(array=w248, index=1) -> (element=w249:cluster{string[]})
                n159 = call <vilib>:"NT Read String.vi"("name"=w251) -> ("value"=w250:string)  [unwired: 8 in, 2 out]
                n160 = Unbundle(w249) -> (w246:string[])
                n161 = Match First String(2:w246, 3:w250) -> (0:w245:i32)  [unwired: 1 out]
                n162 = property on="Test Ring" class="Ring (strict)"("Value"=w245, "Strings []"=w246) -> ()  [unwired: 2 in, 2 out]
                n163 = property on="Test Ring" class="Ring (strict)"("Visible"=TRUE) -> ()  [unwired: 2 in, 2 out]
                n164 = property on="Test Slider" class="Slide (strict)"("Visible"=FALSE) -> ()  [unwired: 2 in, 2 out]
              }
              frame "Exposure  **" {
                n165 = Index Array(array=w257, index=2) -> (element=w258:cluster{string[]})
                n166 = call <vilib>:"NT Read String.vi"("name"=w260) -> ("value"=w259:string)  [unwired: 8 in, 2 out]
                n167 = Unbundle(w258) -> (w254:string[])
                n168 = Match First String(2:w254, 3:w259) -> (0:w255:i32)  [unwired: 1 out]
                n169 = property on="Test Ring" class="Ring (strict)"("Value"=w255, "Strings []"=w254) -> ()  [unwired: 2 in, 2 out]
                n170 = property on="Test Ring" class="Ring (strict)"("Visible"=TRUE) -> ()  [unwired: 2 in, 2 out]
                n171 = property on="Test Slider" class="Slide (strict)"("Visible"=FALSE) -> ()  [unwired: 2 in, 2 out]
              }
              frame "Exposure Priority  **" {
                n172 = Index Array(array=w266, index=3) -> (element=w267:cluster{string[]})
                n173 = call <vilib>:"NT Read String.vi"("name"=w269) -> ("value"=w268:string)  [unwired: 8 in, 2 out]
                n174 = Unbundle(w267) -> (w263:string[])
                n175 = Match First String(2:w263, 3:w268) -> (0:w264:i32)  [unwired: 1 out]
                n176 = property on="Test Ring" class="Ring (strict)"("Value"=w264, "Strings []"=w263) -> ()  [unwired: 2 in, 2 out]
                n177 = property on="Test Ring" class="Ring (strict)"("Visible"=TRUE) -> ()  [unwired: 2 in, 2 out]
                n178 = property on="Test Slider" class="Slide (strict)"("Visible"=FALSE) -> ()  [unwired: 2 in, 2 out]
              }
              frame "Color Enable  **" {
                n179 = Index Array(array=w275, index=4) -> (element=w276:cluster{string[]})
                n180 = call <vilib>:"NT Read String.vi"("name"=w278) -> ("value"=w277:string)  [unwired: 8 in, 2 out]
                n181 = Unbundle(w276) -> (w272:string[])
                n182 = Match First String(2:w272, 3:w277) -> (0:w273:i32)  [unwired: 1 out]
                n183 = property on="Test Ring" class="Ring (strict)"("Value"=w273, "Strings []"=w272) -> ()  [unwired: 2 in, 2 out]
                n184 = property on="Test Ring" class="Ring (strict)"("Visible"=TRUE) -> ()  [unwired: 2 in, 2 out]
                n185 = property on="Test Slider" class="Slide (strict)"("Visible"=FALSE) -> ()  [unwired: 2 in, 2 out]
              }
              frame Default {
                n186 = property on="Test Ring" class="Ring (strict)"("Visible"=FALSE) -> ()  [unwired: 2 in, 2 out]
                n187 = property on="Test Slider" class="Slide (strict)"("Visible"=FALSE) -> ()  [unwired: 2 in, 2 out]
              }
              frame "Brightness  **", "Color Level  **", "Compression  **", "FPS  **", "Sharpness  **" {
                n188 = call <vilib>:"NT Read Number.vi"("name"=w284) -> ("value"=w283:dbl)  [unwired: 8 in, 2 out]
                n189 = local write "Test Slider"(w283) -> ()
                n190 = property on="Test Slider" class="Slide (strict)"("Visible"=TRUE, "Scale.Maximum"=100.0 ("Scale.Range:Maximum")) -> ()  [unwired: 2 in, 2 out]
                n191 = property on="Test Ring" class="Ring (strict)"("Visible"=FALSE) -> ()  [unwired: 2 in, 2 out]
              }
            }
          }
        }
        n192 = property on="Progress" class="Clust (strict)"("Visible"=FALSE) -> ()  [unwired: 2 in, 2 out]
      }
      event "Test Name": Mouse Enter {
        # "Populate the ring with the list of tests"
        n193 = event-data() -> ()  [unwired: 1 in, 1 out]
        n194 = call <vilib>:"NT Read String Array.vi"("name"="TestMode/TestList" ("Name")) -> ("value"=w291:string[])  [unwired: 8 in, 2 out]
        n195 = Build Array (concatenate)("Select the test to run...", w291) -> (w290:string[])
        n196 = property on="Test Name" class="Ring (strict)"("Strings []"=w290) -> ()  [unwired: 2 in, 2 out]
      }
      event "Test Name": Value Change {
        w292 = FALSE ("Visible")
        # "Tell the robot the test name to run"
        n197 = event-data() -> ("NewVal"=w296:u16)  [unwired: 1 in]
        n198 = property on="Test Name" class="Ring (strict)"() -> ("Strings []"=w297:string[])  [unwired: 2 in, 2 out]
        n199 = local write "Progress"(T5 {"Test Progress"=0, "Test Progress Text"=""} ("Progress")) -> ()
        n200 = Index Array(array=w297, index=w296) -> (element=w295:string)
        n201 = call <vilib>:"NT Write String.vi"("value"=w295, "name"="TestMode/TestName" ("Name")) -> ()  [unwired: 9 in, 1 out]
        n202 = property on="Progress" class="Clust (strict)"("Visible"=TRUE) -> ()  [unwired: 2 in, 2 out]
        n203 = property on="Motor" class="Clust (strict)"("Visible"=w292) -> ()  [unwired: 2 in, 2 out]
        n204 = property on="Test Slider" class="Slide (strict)"("Visible"=w292) -> ()  [unwired: 2 in, 2 out]
        n205 = property on="On/Off" class="Bool (strict)"("Visible"=w292) -> ()  [unwired: 2 in, 2 out]
        n206 = property on="Rev/Fwd" class="Clust (strict)"("Visible"=w292) -> ()  [unwired: 2 in, 2 out]
        n207 = property on="Test Ring" class="Ring (strict)"("Visible"=w292) -> ()  [unwired: 2 in, 2 out]
      }
      event "Select Auto": Mouse Enter {
        # "Populate the combo box with the list of autonomous options"
        n208 = event-data() -> ()  [unwired: 1 in, 1 out]
        n209 = call <vilib>:"NT Read String Array.vi"("name"="Auto List" ("Name")) -> ("value"=w299:string[])  [unwired: 8 in, 2 out]
        n210 = property on="Select Auto" class="CmbBox"("Strings[]"=w299) -> ()  [unwired: 2 in, 2 out]
      }
      event "Select Auto": Value Change {
        # "User modified the Auto Selection. Write to NT variable so robot knows."
        n211 = event-data() -> ("NewVal"=w301:string)  [unwired: 1 in]
        n212 = call <vilib>:"NT Write String.vi"("value"=w301, "name"="Auto Selector" ("Name")) -> ()  [unwired: 9 in, 1 out]
      }
      event "CheckList": Double Click {
        # "Shift clears all"
        # "Update symbols on the listbox"
        n213 = event-data() -> ("PlatMods.Shift"=w303:bool, "Row"=w305:i32)  [unwired: 1 in]
        n214 = case shown="True" w303 {
          tunnel: w305 -> [w309 _]
          tunnel: 1 -> [w308 _]
          frame False {
            n215 = property on="CheckList" class="LstBox (strict)"() -> ("Item Symbols"=w307:i32[])  [unwired: 2 in, 2 out]
            n216 = Replace Array Subset(array=w307, new element=w308, index=w309) -> (w306:i32[])
            n217 = property on="CheckList" class="LstBox (strict)"("Item Symbols"=w306) -> ()  [unwired: 2 in, 2 out]
          }
          frame True {
            w310 = 0 ("Top Row")
            n218 = property on="CheckList" class="LstBox (strict)"() -> ("Number of Rows"=w312:u32)  [unwired: 2 in, 2 out]
            n219 = Initialize Array(0, w312) -> (w311:i32[])
            n220 = property on="CheckList" class="LstBox (strict)"("Top Row"=w310, "Value"=w310, "Item Symbols"=w311) -> ()  [unwired: 2 in, 2 out]
          }
        }
      }
      event "CheckList": Key Down {
        # "Update symbols on the listbox\nLeft and right keys check and uncheck"
        n221 = event-data() -> ("VKey"=w315:T20)  [unwired: 1 in]
        n222 = case shown="\"Left\", \"Right\"" w315 {
          selector: w315 -> [w320 _]
          tunnel: eventvkey."Left" ("VKey") -> [w318 _]
          frame "Left", "Right" {
            n223 = Equal?(x=w318, y=w320) -> (x = y?=w319:bool)
            n224 = Select(t=0, s=w319, f=1) -> (s? t:f=w321:i32)
            n225 = property on="CheckList" class="LstBox (strict)"() -> ("Item Symbols"=w324:i32[])  [unwired: 2 in, 2 out]
            n226 = Replace Array Subset(array=w324, new element=w321, index="CheckList") -> (w323:i32[])
            n227 = property on="CheckList" class="LstBox (strict)"("Item Symbols"=w323) -> ()  [unwired: 2 in, 2 out]
          }
          frame Default {
          }
        }
      }
      event "Motor.Enable": Value Change {
        # "When the test mode otor enable helper is set, update that\ntree row item's value"
        n228 = event-data() -> ("NewVal"=w329:bool)  [unwired: 1 in]
        n229 = Unbundle("Motor") -> ("Value"=w328:dbl)  [unwired: 1 out]
        n230 = Select(t=w328, s=w329, f=0.0) -> (s? t:f=w326:dbl)
        n231 = call <vilib>:"NT Write Number.vi"("value"=w326, "name"=w325) -> ()  [unwired: 9 in, 1 out]
      }
      event "Test Slider": Value Change {
        # "When the test mode slider helper is set, update that\ntree row item's value"
        n232 = event-data() -> ("NewVal"=w331:dbl)  [unwired: 1 in]
        n233 = call <vilib>:"NT Write Number.vi"("value"=w331, "name"=w332) -> ()  [unwired: 9 in, 1 out]
      }
      event "On/Off": Value Change {
        # "When the test mode on/off helper value is set, update that\ntree row item's value"
        n234 = event-data() -> ("NewVal"=w335:bool)  [unwired: 1 in]
        n235 = Boolean To (0,1)(Boolean=w335) -> (0, 1=w334:i16)
        n236 = call <vilib>:"NT Write Number.vi"("value"=w334, "name"=w333) -> ()  [unwired: 9 in, 1 out]
      }
      event "Rev/Fwd": Value Change {
        # "When the test mode helper value for relays is set, update that\ntree row item's value"
        n237 = event-data() -> ("NewVal.Forward"=w342:bool, "NewVal.Reverse"=w341:bool)  [unwired: 1 in]
        n238 = Boolean To (0,1)(Boolean=w342) -> (0, 1=w338:i16)
        n239 = Boolean To (0,1)(Boolean=w341) -> (0, 1=w340:i16)
        n240 = Negate(x=w340) -> (-x=w339:i16)
        n241 = Add(x=w338, y=w339) -> (x+y=w337:i16)
        n242 = call <vilib>:"NT Write Number.vi"("value"=w337, "name"=w336) -> ()  [unwired: 9 in, 1 out]
      }
      event "Test Ring": Value Change {
        # "When a test mode helper value is selected from the ring,\nset the tree item's variable to the string value"
        n243 = event-data() -> ("NewVal"=w345:u16)  [unwired: 1 in]
        n244 = property on="Test Ring" class="Ring (strict)"() -> ("Strings []"=w346:string[])  [unwired: 2 in, 2 out]
        n245 = Index Array(array=w346, index=w345) -> (element=w344:string)
        n246 = call <vilib>:"NT Write String.vi"("value"=w344, "name"=w343) -> ()  [unwired: 9 in, 1 out]
      }
      event "Rec Mode": Value Change {
        # "Update globals for recording mode and path to read log from.\nClear when logging and let NetworkTables set path for vision to\nuse."
        n247 = event-data() -> ("NewVal"=w355:enum32{"Stop", "Record", "Playback"})  [unwired: 1 in]
        n248 = global write "WPI_DashboardLogging Global.vi" "Logging Filename"(path "") -> ()
        n249 = global write "WPI_DashboardLogging Global.vi" "Recording"(w355) -> ()
        n250 = case shown="\"Playback\"" w355 {
          tunnel: w354 -> [_ w357 w365]
          tunnel: [_ _ w364] -> w352
          tunnel: [_ _ w363] -> _
          tunnel: w350 -> [_ _ w361]
          tunnel: cluster{i32, i32} {-250, 170} -> [_ _ w360]
          tunnel: [_ _ T21 {"Image Size"=TRUE, "Image Type"=TRUE, "Pixel Value"=TRUE, "ROI Information"=TRUE, "Zoom Factor"=FALSE} ("Image Information Shown:All Elements")] -> w347
          tunnel: [_ _ TRUE ("Zoom Factor")] -> w348
          frame Default {
          }
          frame "Stop", "Record" {
            # "Place Window too"
            n251 = invoke class="VI" method="FP.Close"(reference=w357) -> (reference out=w356:refnum<vi>)  [unwired: 2 in, 2 out]
            n252 = invoke class="VI" method="Abort VI"(reference=w356) -> ()  [unwired: 2 in, 3 out]
          }
          frame "Playback" {
            n253 = call "Open Playback Panel.vi"("Offset"=w360, "DB VI Ref"=w361, "Playback in"=w365) -> ("Playback out"=w362:refnum<vi>)  [unwired: 8 in]
            n254 = register-events(w362) -> (reference out=w364:refnum<event-registration>, error out=w363:errorcluster)  [unwired: 2 in]
          }
        }
        n255 = property on="Camera Image Right" class="ImageControl"("Image Information Shown"=w347, "Image Information Visible"=w348) -> ()  [unwired: 2 in, 2 out]
        n256 = property on="Camera Image" class="ImageControl"("Image Information Shown"=w347, "Image Information Visible"=w348) -> ()  [unwired: 2 in, 2 out]
        n257 = call <vilib>:"WPI_DashboardNT Log FieldName Cache.vi"("Operation"=enum16{"Lookup/Add", "Index", "Clear"}."Clear") -> ()  [unwired: 8 in, 3 out]
      }
      event Panel Close {
        w366 = enum32{"Stop", "Record", "Playback"}."Stop" ("Rec Mode")
        # "Playback window has been closed, abort"
        n258 = event-data() -> ()  [unwired: 1 in, 4 out]
        n259 = local write "Rec Mode"(w366) -> ()
        n260 = global write "WPI_DashboardLogging Global.vi" "Recording"(w366) -> ()
      }
      event Panel Close {
        # "Abort playback window and ourself"
        n261 = event-data() -> ()  [unwired: 1 in, 4 out]
        n262 = invoke class="VI" method="FP.Close"(reference=w369) -> (reference out=w368:refnum<vi>)  [unwired: 2 in, 2 out]
        n263 = invoke class="VI" method="Abort VI"(reference=w368) -> (error out=w367:errorcluster)  [unwired: 2 in, 2 out]
        n264 = invoke class="VI" method="Abort VI"(error in=w367) -> ()  [unwired: 2 in, 3 out]
      }
      event "Tree": Double Click {
        n265 = event-data() -> ("PlatMods"=w375:T23, "Tag"=w372:string)  [unwired: 1 in]
        n266 = Unbundle(w375) -> ("Shift"=w374:bool)  [unwired: 4 out]
        n267 = String Subset(string=w372, length (rest)=1 ("length (rest)")) -> (substring=w371:string)  [unwired: 1 in]
        n268 = Not(x=w374) -> (.not. x?=w373:bool)
        n269 = case shown="\"/\"" w371 {
          tunnel: w372 -> [_ w377]
          tunnel: w373 -> [_ w376]
          frame Default {
          }
          frame "/" {
            n270 = call <vilib>:"NT Update Persistence.vi"("Persistence"=w376, "Name"=w377) -> ()  [unwired: 9 in, 1 out]
          }
        }
      }
    }
  }
  n271 = while {
    tunnel: w54 -> [w379]
    i -> [w382]
    stop <- FALSE stop-if-true
    n272 = Wait (ms)(milliseconds to wait=u32 100) -> ()  [unwired: 1 out]
    n273 = case shown="\"Playback\"" "Rec Mode" {
      tunnel: w382 -> [_ _ w397]
      tunnel: [u32 2829099 ("Base Color") u32 11141120 ("Target Color") w386] -> w378
      frame "Stop", Default {
        # "Reset the color, extra updates don't cost much"
      }
      frame "Record" {
      }
      frame "Playback" {
        # "Playback"
        n274 = Quotient & Remainder(x=w397, y=u32 50 ("milliseconds to wait")) -> (x-y*floor(x/y)=w393:u32)  [unwired: 1 out]
        n275 = Divide(x=w393, y=u32 50 ("milliseconds to wait")) -> (x/y=w390:dbl)
        n276 = Multiply(x=6.283185307179586, y=w390) -> (x*y=w395:dbl)
        n277 = Sine(x=w395) -> (sin(x)=w394:dbl)
        n278 = Absolute Value(x=w394) -> (abs(x)=w387:dbl)
        n279 = call "Interpolate RGB Color.vi"("Proportion"=w387, "Target Color"=u32 30976, "Base Color"=u32 2829099) -> ("Result Color"=w386:u32)  [unwired: 8 in]
      }
    }
    n280 = property class="Pane"(reference=w379, "PaneColor"=w378) -> ()  [unwired: 1 in, 2 out]
  }
  n281 = local write "Dashboard Tab"(T2."Drive" ("Dashboard Tab")) -> ()
  n282 = property on="On/Off" class="Bool (strict)"("Visible"=w26) -> ()  [unwired: 2 in, 2 out]
  n283 = property on="Motor" class="Clust (strict)"("Visible"=w26) -> ()  [unwired: 2 in, 2 out]
  n284 = property on="Progress" class="Clust (strict)"("Visible"=w26) -> ()  [unwired: 2 in, 2 out]
  n285 = property on="Test Ring" class="Ring (strict)"("Visible"=w26) -> ()  [unwired: 2 in, 2 out]
  n286 = property on="Rev/Fwd" class="Clust (strict)"("Visible"=w26) -> ()  [unwired: 2 in, 2 out]
  n287 = while {
    tunnel: u16 1741 ("timeout ms (25000)") -> [w399]
    stop <- FALSE stop-if-true
    n288 = TCP Create Listener(10:w399) -> (0:w398:errorcluster, 3:w400:refnum<k5>)  [unwired: 4 in, 1 out]
    n289 = case shown="No Error" w398 {
      selector: w398 -> [w402 _]
      tunnel: w400 -> [w403 _]
      frame No Error {
        n290 = while {
          tunnel: w403 -> [w406]
          tunnel: w402 -> [w405]
          stop <- FALSE stop-if-true
          n291 = TCP Wait On Listener(8:w405, 11:w406) -> (0:w407:errorcluster, 4:w408:refnum<k5>)  [unwired: 2 in, 3 out]
          n292 = local write "TCP"(w408) -> ()
          n293 = case shown="Error" w407 {
            frame No Error {
            }
            frame Error {
              n294 = Wait (ms)(milliseconds to wait=u32 1000) -> ()  [unwired: 1 out]
            }
          }
        }
      }
      frame Error {
        n295 = Wait (ms)(milliseconds to wait=u32 1000) -> ()  [unwired: 1 out]
      }
    }
  }
  n296 = global write "WPI_DashboardLogging Global.vi" "Recording"(w49) -> ()
  n297 = local write "Rec Mode"(w49) -> ()
  n298 = call <vilib>:"NT Write String.vi"("value"="Select Auto", "name"="Auto Selector" ("Name")) -> ()  [unwired: 9 in, 1 out]
